vi "Simple Reader.vi"(8 "error in (no error)":errorcluster, 11 "Andeen-Hagerling Driver in":refnum<class "Andeen-Hagerling Driver.lvclass">) -> (0 "error out":errorcluster, 2 "Signals":dbl[](array[numeric]), 3 "Andeen-Hagerling Driver out":refnum<class "Andeen-Hagerling Driver.lvclass">)   [LabVIEW 2016, in "Andeen-Hagerling Driver.lvclass"]
uses:
  Andeen-Hagerling Driver.lvclass
  D:/github/NHMFL_Core/Libraries/Instruments/VISA Instrument/VISA Instrument.lvclass
  VISA Instrument/VISA Instrument.lvclass/VISA Instrument.ctl
  VISA Instrument/Read VISA resource.vi
  VISA Instrument/Write VISA resource.vi
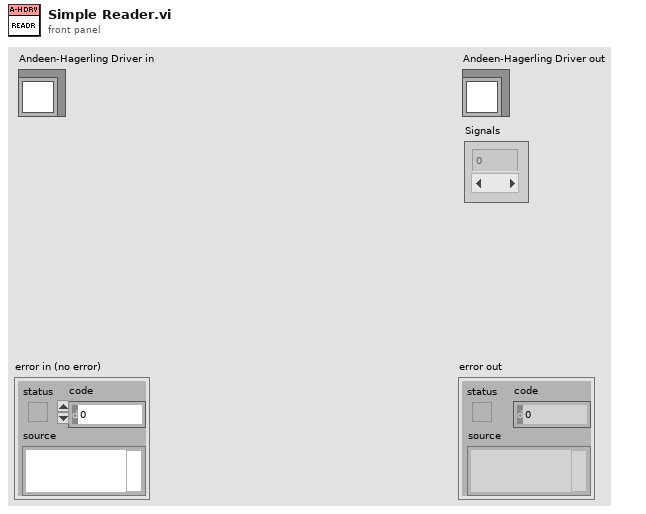
[diagram p1: front panel]
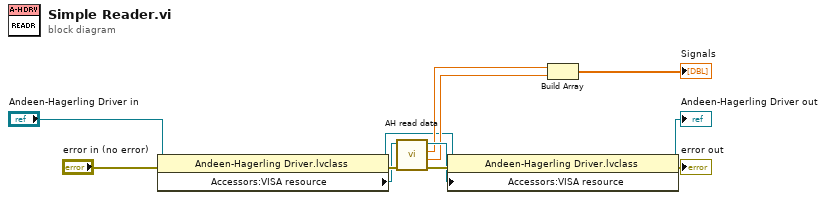
[diagram p0: block diagram]
diagram:
  n1 = property class="Andeen-Hagerling Driver.lvclass"(reference="Andeen-Hagerling Driver in", error in="error in (no error)") -> (reference out=w6:refnum<class "Andeen-Hagerling Driver.lvclass">, error out=w11:errorcluster, "Accessors:VISA resource"=w7:refnum<visa-resource-name>)
  n2 = call "AH read data.vi"("error in (no error)"=w11, "VISA Resource Name"=w7) -> ("error out"=w12:errorcluster, "Loss"=w9:dbl, "Capacitance"=w8:dbl, "VISA Resource Name Out"=w10:refnum<visa-resource-name>)  [unwired: 6 in]
  n3 = property class="Andeen-Hagerling Driver.lvclass"(reference=w6, error in=w12, "Accessors:VISA resource"=w10) -> (reference out=→"Andeen-Hagerling Driver out":refnum<class "Andeen-Hagerling Driver.lvclass">, error out=→"error out":errorcluster)
  n4 = Build Array(w8, w9) -> (→"Signals":dbl[])
